vi "MatchRegExStd.vi"(5 "capture index":i32, 7 "Options":cluster{"Compile":u32, "Match":u32} {"Match" format="%.0x"; "Compile" format="%.0x"}, 8 "error in":errorcluster, 9 "offset (0)":i32, 10 "search pattern":string, 11 "string":string) -> (0 "error out":errorcluster, 1 "after substring":string, 2 "match substring":string, 3 "before substring":string, 4 "offset past match":i32, 6 "match offset":i32)   [LabVIEW 2021, in "libpcre2-8.lvlib"]
uses:
  libpcre2-8.lvlib
  Pcre2GetOvectorPointer8.vi
  Pcre2MoOfSubstrNumFmOv.vi
  Pcre2CompileError.vi
  Pcre2ErrorNull.vi
  Pcre2LibError.vi
  Pcre2FnkCallError.vi
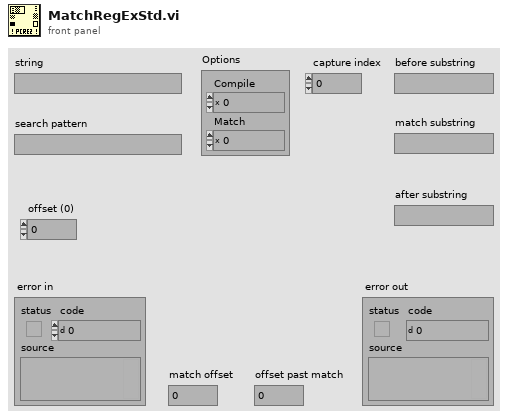
[diagram p1: front panel]
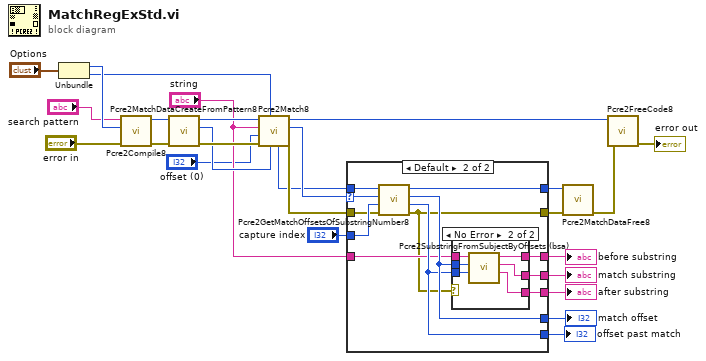
[diagram p0: block diagram]
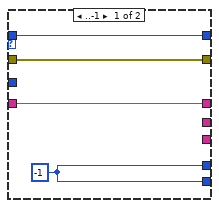
[diagram p2: hidden frame]
diagram:
  n1 = Unbundle("Options") -> ("Compile"=w11:u32, "Match"=w10:u32)
  n2 = call "Pcre2Compile8.vi"("error in"="error in", "Options"=w11, "Pattern"="search pattern") -> ("error out"=w18:errorcluster, "pCode"=w17:u64)  [unwired: 7 in]
  n3 = call "Pcre2MatchDataCreateFromPattern8.vi"("error in"=w18, "pCode"=w17) -> ("error out"=w19:errorcluster, "pMatchData"=w5:u64, "pCode"=w20:u64)  [unwired: 7 in]
  n4 = call "Pcre2Match8.vi"("pMatchData"=w5, "Options"=w10, "error in"=w19, "StartOffset"="offset (0)", "Subject"="string", "pCode"=w20) -> ("error out"=w9:errorcluster, "MatchResult"=w14:i32, "pCode"=w16:u64, "pMatchData"=w6:u64)  [unwired: 2 in]
  n5 = case shown="Default" w14 {
    selector: w14 -> [_ w32]
    tunnel: w6 -> [w30 w42]
    tunnel: [w28 w41] -> w26
    tunnel: [_ w40] -> w25
    tunnel: [_ w39] -> w24
    tunnel: [w30 w38] -> w8
    tunnel: [w27 w37] -> w23
    tunnel: [w27 w36] -> w22
    tunnel: "string" -> [w28 w35]
    tunnel: "capture index" -> [_ w34]
    tunnel: w9 -> [w29 w31]
    tunnel: [w29 w33] -> w7
    frame ..-1 {
      w27 = -1 ("MatchOffset")
    }
    frame Default {
      n6 = call "Pcre2GetMatchOffsetsOfSubstringNumber8.vi"("error in"=w31, "Number"=w34, "MatchResult"=w32, "pMatchData"=w42) -> ("error out"=w33:errorcluster, "OffsetPastMatch"=w36:i32, "MatchOffset"=w37:i32, "pMatchData"=w38:u64)  [unwired: 4 in]
      n7 = case shown="No Error" w33 {
        tunnel: [w43 w46] -> w41
        tunnel: [_ w44] -> w40
        tunnel: [_ w45] -> w39
        tunnel: w37 -> [_ w48]
        tunnel: w36 -> [_ w47]
        tunnel: w35 -> [w43 w49]
        frame Error {
        }
        frame No Error {
          n8 = call "Pcre2SubstringFromSubjectByOffsets (bsa).vi"("OffsetPastMatch"=w47, "MatchOffset"=w48, "Subject"=w49) -> ("AfterSubstring"=w44:string, "Substring"=w45:string, "BeforeSubstring"=w46:string)  [unwired: 6 in]
        }
      }
    }
  }
  "match offset" <- w23
  "offset past match" <- w22
  "before substring" <- w26
  "match substring" <- w24
  "after substring" <- w25
  n9 = call "Pcre2MatchDataFree8.vi"("error in"=w7, "pMatchData"=w8) -> ("error out"=w15:errorcluster)  [unwired: 9 in]
  n10 = call "Pcre2FreeCode8.vi"("error in"=w15, "pCode"=w16) -> ("error out"=→"error out":errorcluster)  [unwired: 9 in]
